vi "Filament.vi"(0 "Strings in":string[](array[string]), 1 "Dubs in":dbl[](array[numeric])) -> ()   [LabVIEW 2018]
panel:
  in  "Enable":dbl
  in  "Filament current (A)":dbl=0.3
  in  "Burn time (s)":dbl=10.0
  in  "subvi":bool=TRUE
  in  "Filament File":path=path "C:/CuspControl/GPIB and Network/Cusp/esourceRampVoltandState.txt"
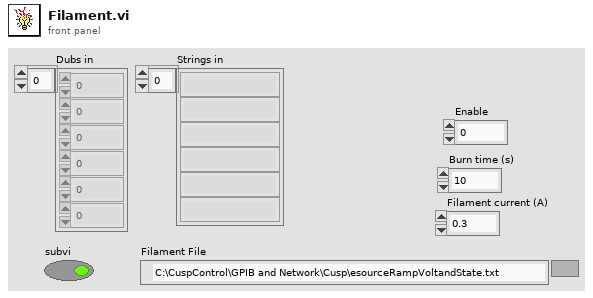
[diagram p1: front panel]
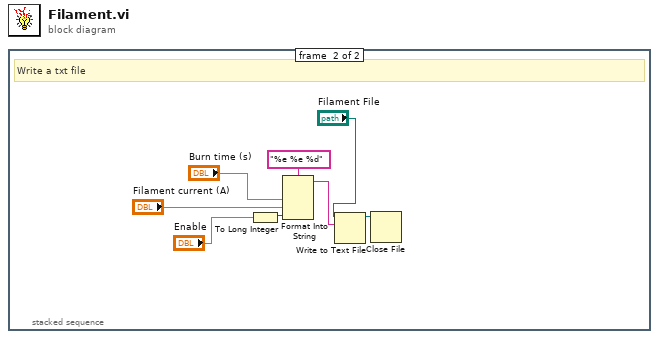
[diagram p0: block diagram]
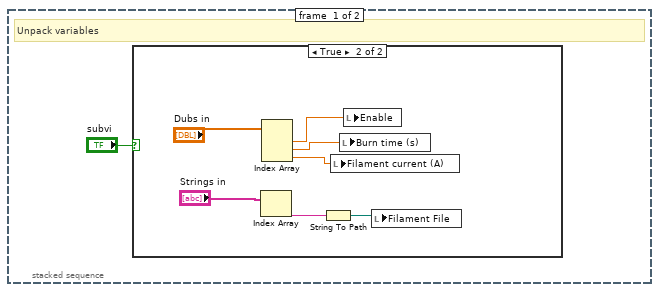
[diagram p2: hidden frame]
diagram:
  n1 = stacked-sequence {
    frame #0 {
      # "Unpack variables"
      n2 = case shown="True" "subvi" {
        frame False {
        }
        frame True {
          n3 = Index Array(array="Strings in") -> (element=w6:string)  [unwired: 1 in]
          n4 = Index Array(array="Dubs in") -> (element #1=w2:dbl, element #2=w4:dbl, element #3=w3:dbl)  [unwired: 3 in]
          n5 = String To Path(string=w6) -> (path=w5:path)
          n6 = local write "Filament current (A)"(w3) -> ()
          n7 = local write "Burn time (s)"(w4) -> ()
          n8 = local write "Enable"(w2) -> ()
          n9 = local write "Filament File"(w5) -> ()
        }
      }
    }
    frame #1 {
      # "Write a txt file"
      n10 = To Long Integer(number="Enable") -> (32bit integer=w13:i32)
      n11 = Format Into String(format string="%e %e %d", "Burn time (s)", "Filament current (A)", w13) -> (resulting string=w16:string)  [unwired: 2 in, 1 out]
      n12 = Write to Text File(file (use dialog)="Filament File", text=w16) -> (refnum out=w15:refnum<file>)  [unwired: 2 in, 2 out]
      n13 = Close File(refnum=w15) -> ()  [unwired: 1 in, 2 out]
    }
  }
